vi "New Card Set Up.vi"(10 "Card Cluster":T1) -> (0 "Measurement Time 2":dbl, 1 "Card chosen":i32, 2 "Warm Up Time 2":dbl, 3 "Continuous?":bool, 4 "V Range (12: 1000) 2":u16(ring)=9 items=["AUTO", "1.5", "3", "6", "10", "15", "30", "60", "100", "150", "300", "600", "1000"], 5 "A Range (9: 5A) 2":u16(ring)=9 items=["AUTO", "10 mA", "20 mA", "50 mA", "100 mA", "200 mA", "500 mA", "1 A", "2 A", "5 A", "10 A", "20 A", "50 A", "S-AUTO", "50 mV", "100 mV", "250 mV", "500 mV", "1 V", "2.5 V", "5 V", "10 V"])   [LabVIEW 2013, in "Universal Power Meter.lvlib" / "WT1600.lvlib" / "WT1600.lvclass"]
uses:
  WT1600.lvclass
panel:
  in  "V Range (12: 1000)":u16(ring)=9 items=["AUTO", "1.5", "3", "6", "10", "15", "30", "60", "100", "150", "300", "600", "1000"]
  in  "A Range (9: 5A)":u16(ring)=9 items=["AUTO", "10 mA", "20 mA", "50 mA", "100 mA", "200 mA", "500 mA", "1 A", "2 A", "5 A", "10 A", "20 A", "50 A", "S-AUTO", "50 mV", "100 mV", "250 mV", "500 mV", "1 V", "2.5 V", "5 V", "10 V"]
  in  "Warm Up Time":dbl format="%<%H:%M:%S>t"
  in  "Measurement Time":dbl format="%<%H:%M:%S>t"
  in  "Measurement":enum32{"Continuous", "Timed"}(radio)
  in  "Card to Start":u16(ring) items=["1", "2", "3", "4", "5", "6"]
  in  "Play Button":bool
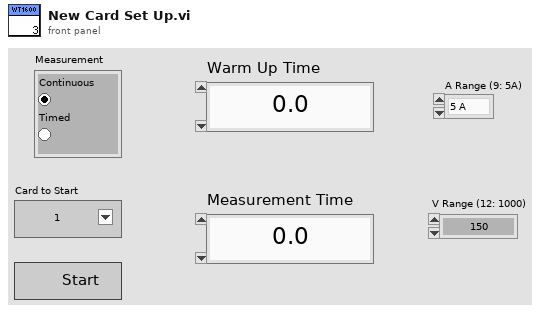
[diagram p1: front panel]
types:
  T1 = cluster{"Card 1":bool, "Card 2":bool, "Card 3":bool, "Card 4":bool, "Card 5":bool, "Card 6":bool}
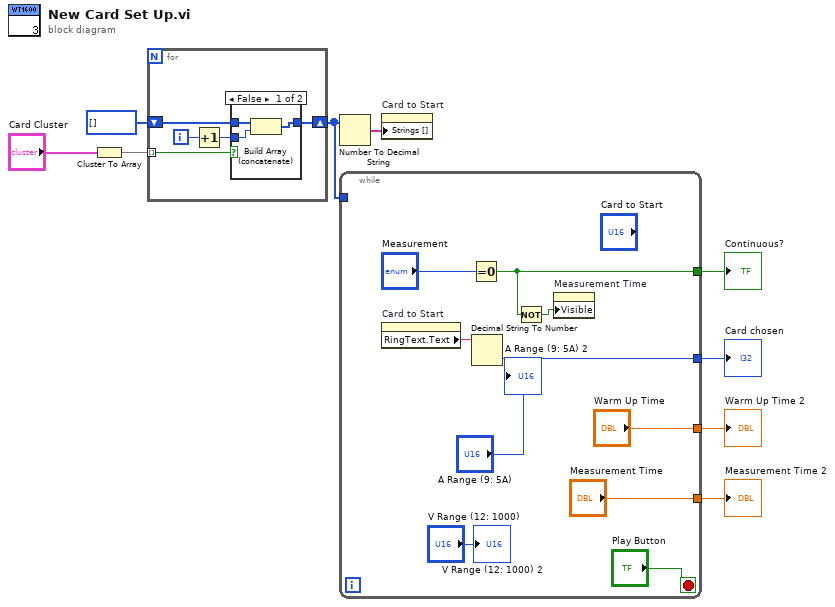
[diagram p0: block diagram]
diagram:
  n1 = Cluster To Array(cluster="Card Cluster") -> (array=w8:bool[])
  n2 = for {
    tunnel: w8 -> [w14] mode=indexing
    shift-right: [w10] -> w6
    shift-left: i32[] [] -> [w13]
    i -> [w12]
    n3 = Increment(x=w12) -> (x+1=w11:i32)
    n4 = case shown="False" w14 {
      tunnel: w13 -> [w17 w18]
      tunnel: w11 -> [w16 _]
      tunnel: [w15 w18] -> w10
      frame False {
        n5 = Build Array (concatenate)(w17, w16) -> (w15:i32[])
      }
      frame True {
      }
    }
  }
  n6 = Number To Decimal String(number=w6) -> (decimal integer string=w5:string[])  [unwired: 1 in]
  n7 = while {
    tunnel: w6 -> [_]
    tunnel: [w26] -> w4
    tunnel: ["Measurement Time"] -> w3
    tunnel: ["Warm Up Time"] -> w2
    tunnel: [w22] -> w1
    stop <- "Play Button" stop-if-true
    n8 = property on="Card to Start" class="Ring (strict)"() -> ("RingText.Text"=w27:string)  [unwired: 2 in, 2 out]
    n9 = Equal To 0?(x="Measurement") -> (x = 0?=w22:bool)
    n10 = Decimal String To Number(string=w27) -> (number=w26:i32)  [unwired: 2 in, 1 out]
    n11 = Not(x=w22) -> (.not. x?=w21:bool)
    n12 = property on="Measurement Time" class="DigNum (strict)"("Visible"=w21) -> ()  [unwired: 2 in, 2 out]
    "A Range (9: 5A) 2" <- "A Range (9: 5A)"
    "V Range (12: 1000) 2" <- "V Range (12: 1000)"
  }
  "Card chosen" <- w4
  "Measurement Time 2" <- w3
  "Warm Up Time 2" <- w2
  "Continuous?" <- w1
  n13 = property on="Card to Start" class="Ring (strict)"("Strings []"=w5) -> ()  [unwired: 2 in, 2 out]
